vi "Discover Nodes.vi"(8 "Error In":errorcluster, 11 "ICommunicate":refnum<class "ICommunicate.lvclass">) -> (0 "Error Out":errorcluster)   [LabVIEW 2024, in "Network Mangement.lvclass"]
uses:
  Network Mangement.lvclass
  HAL/Source/Interfaces/ICommunicate/ICommunicate.lvclass
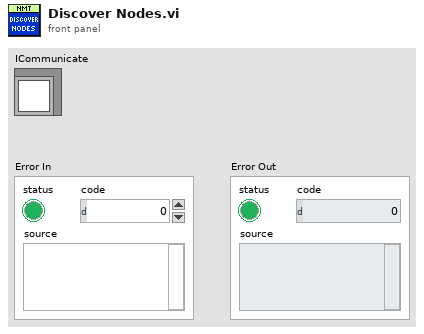
[diagram p1: front panel]
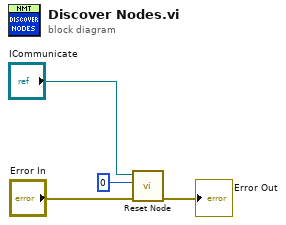
[diagram p0: block diagram]
diagram:
  n1 = call "Reset Node.vi"("Error In"="Error In", "Node-ID"=u8 0, "ICommunicate"="ICommunicate") -> ("Error Out"=→"Error Out":errorcluster)  [unwired: 8 in]
